vi "Analog Read - Serial Connection.vi"() -> ()   [LabVIEW 2011, in "LVH-LINX.lvlib"]
doc: "Read one or more analog values from a LINX device using the LINX serial interface."
uses:
  vi.lib/LabVIEW Hacker/LINX/LVH-LINX.lvlib
panel:
  in  "Stop Button":bool
  out "Analog Data":dbl[](graph)
  in  "AI Channel(s)":u8[](array[numeric])=[0, 1, 2]
  in  "Serial Port":refnum<visa-resource-name>
  # "Analog Read Example (Serial Interface)\n\nThis example demonstrates how to read analog input values from a LINX device connected to the host computer via Serial / USB.\n\nInstructions\n1. Select the COM Port associated with the LINX Device.\n2. Select the Analog Channel(s) to read.\n3. Click the Run Arrow."
  # "Analog Values"
  # "LINX Device Settings"
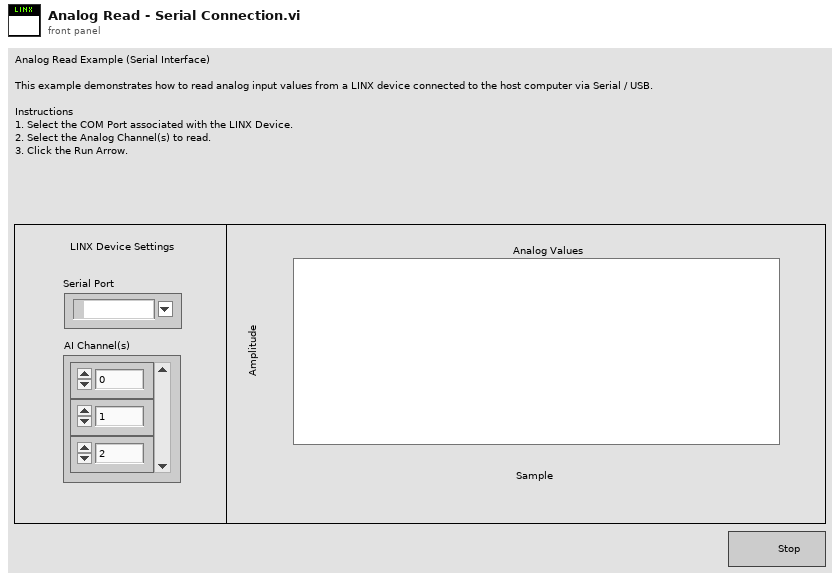
[diagram p1: front panel]
types:
  T1 = typedef "LVH-LINX.lvlib/LINX Ref.ctl" = cluster{"Platform":T2, "Interface":T3, "LINX Device Config":T4}
  T2 = typedef "LVH-LINX.lvlib/Platform.ctl" = enum16{"LINX", "myRIO"}
  T3 = typedef "LVH-LINX.lvlib/Interface.ctl" = enum16{"Serial", "TCP"}
  T4 = typedef "LVH-LINX.lvlib/Device.lvlib/LINX Device Config.ctl" = cluster{"Interface":T3, "COM Port":refnum<visa-resource-name>, "TCP Configuration":T5, "Device Family":T6, "Device ID":u8, "Device Name":string, "TCP Ref":refnum<k5>}
  T5 = typedef "LVH-LINX.lvlib/Device.lvlib/TCP Config.ctl" = cluster{"IP Address":string, "Port":u16}
  T6 = typedef "LVH-LINX.lvlib/Device Family.ctl" = enum8{"National Instruments", "Digilent", "Arduino"}
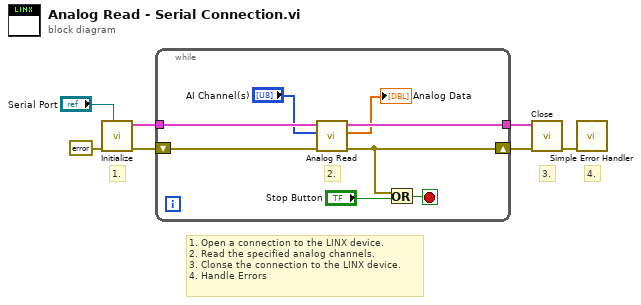
[diagram p0: block diagram]
diagram:
  # "1. Open a connection to the LINX device.\n2. Read the specified analog channels.\n3. Clonse the connection to the LINX device.\n4. Handle Errors"
  # "4."
  # "3."
  # "1."
  n1 = call "Initialize.vi"("Serial Port"="Serial Port", "Error In"=errorcluster {"status"=FALSE, "code"=0, "source"=""}) -> ("Error Out"=w6:errorcluster, "LINX Ref"=w7:T1)  [unwired: 8 in]
  n2 = while {
    tunnel: w7 -> [w15]
    tunnel: [w13] -> w5
    shift-right: [w9] -> w4
    shift-left: w6 -> [w14]
    stop <- w11 stop-if-true
    # "2."
    n3 = call "Analog Read.vi"("Error In"=w14, "AI Channel(s)"="AI Channel(s)", "LINX Resource"=w15) -> ("Error Out"=w9:errorcluster, "Voltages"=→"Analog Data":dbl[], "LINX Resource"=w13:T1)  [unwired: 6 in]
    n4 = Or(x=w9, y="Stop Button") -> (x .or. y?=w11:bool)
  }
  n5 = call "Close.vi"("Error In"=w4, "LINX Resource"=w5) -> ("Error Out"=w2:errorcluster)  [unwired: 8 in, 1 out]
  n6 = call <vilib>:"Simple Error Handler.vi"("error in (no error)"=w2) -> ()  [unwired: 4 in, 5 out]
